vi "fgv_PreChirper Available.vi"(7 "FGV Actions":enum16{"Get", "Set"}(ring), 8 "error in (no error)":errorcluster, 11 "PreChirper Available ? IN":bool) -> (0 "error out":errorcluster, 3 "PreChirper Available ? OUT":bool)   [LabVIEW 2020]
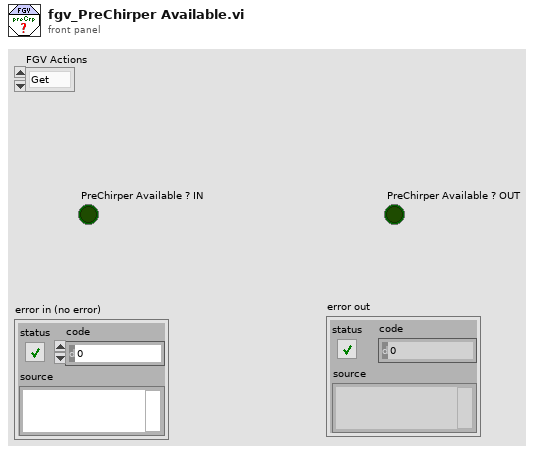
[diagram p1: front panel]
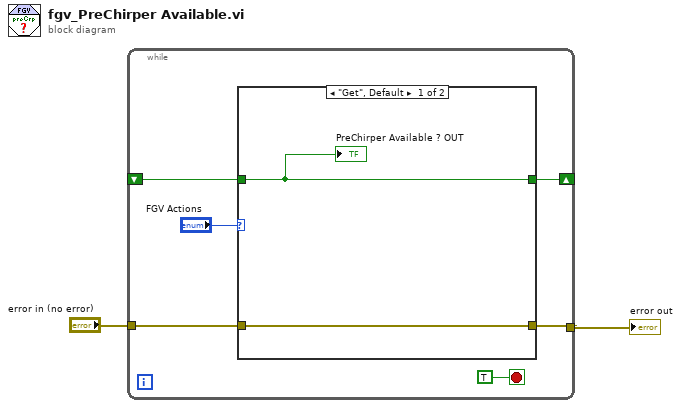
[diagram p0: block diagram]
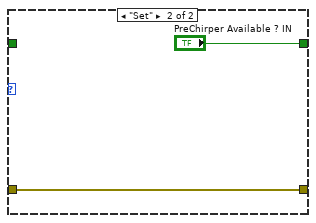
[diagram p2: hidden frame]
diagram:
  n1 = while {
    shift-right: [w6] -> _
    shift-left: _ -> [w5]
    tunnel: "error in (no error)" -> [w4]
    tunnel: [w3] -> w1
    stop <- TRUE stop-if-true
    n2 = case shown="\"Get\", Default" "FGV Actions" {
      tunnel: [w10 "PreChirper Available ? IN"] -> w6
      tunnel: w5 -> [w10 _]
      tunnel: w4 -> [w9 w11]
      tunnel: [w9 w11] -> w3
      frame "Get", Default {
        "PreChirper Available ? OUT" <- w10
      }
      frame "Set" {
      }
    }
  }
  "error out" <- w1
